vi "Check if Session Exists.vi"(8 "error in (no error)":errorcluster, 11 "Web Request in":refnum<class "Web Request.lvclass">) -> (0 "error out":errorcluster, 2 "Logged in?":bool, 3 "Web Request out":refnum<class "Web Request.lvclass">)   [LabVIEW 2016, in "WSsupport.lvlib"]
uses:
  WSsupport.lvlib
  <vilib>/wsapi/Web Request.lvclass
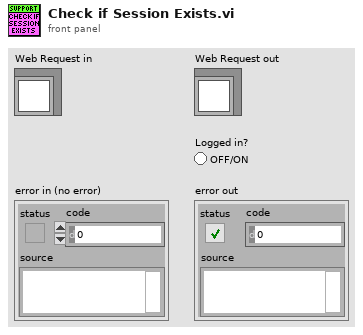
[diagram p1: front panel]
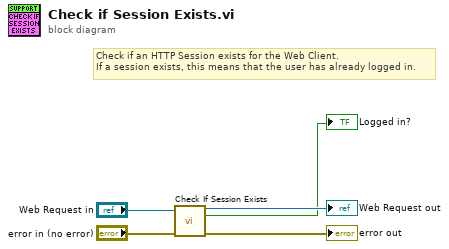
[diagram p0: block diagram]
diagram:
  # "Check if an HTTP Session exists for the Web Client.\nIf a session exists, this means that the user has already logged in."
  n1 = call <vilib>:"Check If Session Exists.vi"("LabVIEW Web Service Request"="Web Request in", "error in (no error)"="error in (no error)") -> ("LabVIEW Web Service Request out"=→"Web Request out":refnum<class "Web Request.lvclass">, "session exists?"=→"Logged in?":bool, "error out"=→"error out":errorcluster)  [unwired: 11 in]
